vi "BLAS3 Utility.vi"   [LabVIEW 2020, in "NI_AALBLAS.lvlib"]
uses:
  <vilib>/Analysis/NI_AALBLAS.lvlib
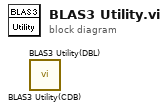
[diagram p0: block diagram]
diagram:
  n1 = call <vilib>:"BLAS3 Utility(CDB).vi"() -> ()  [unwired: 14 in, 6 out]
  n2 = call <vilib>:"BLAS3 Utility(DBL).vi"() -> ()  [unwired: 14 in, 6 out]
